vi "IMAQdx Write Attributes To String.vi"(8 "error in":errorcluster, 11 "Session In":T1) -> (0 "error out":errorcluster, 2 "Attributes String Out":string, 3 "Session Out":T1)   [LabVIEW 2020, in "NI_Vision_Acquisition_Software.lvlib"]
doc: "Save current configuration settings for a camera to a string."
uses:
  NI_Vision_Acquisition_Software.lvlib
  IMAQdx.ctl
  niimaqdx.dll
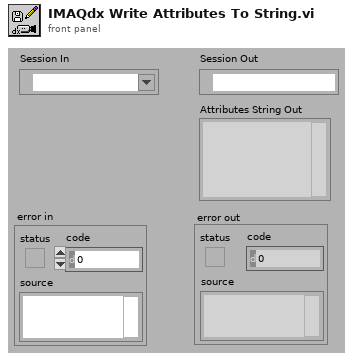
[diagram p1: front panel]
types:
  T1 = typedef "IMAQdx.ctl" = refnum<k21>
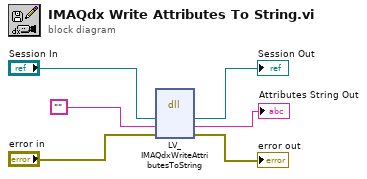
[diagram p0: block diagram]
diagram:
  n1 = dll-call lib="niimaqdx.dll" fn="LV_IMAQdxWriteAttributesToString"("Session In"="Session In", "buffer"="", "error in"="error in") -> ("Session In"=→"Session Out":T1, "buffer"=→"Attributes String Out":string, "error in"=→"error out":errorcluster)  [unwired: 4 in, 2 out]
